vi "Verify Password.vi"(8 "error in (no error)":errorcluster) -> (0 "error out":errorcluster, 3 "Verified?":bool)   [LabVIEW 2017]
uses:
  <vilib>/Utility/sysdir.llb/System Directory Type.ctl
  <vilib>/Utility/config.llb/Write Key (String).vi
  <vilib>/Utility/config.llb/NI_LVConfig.lvlib
panel:
  in  "Verify":string
  in  "Cancel":bool
  in  "Change PWD":bool
  in  "Continue":bool
  in  "Password":string
  # "Administrative Password Management"
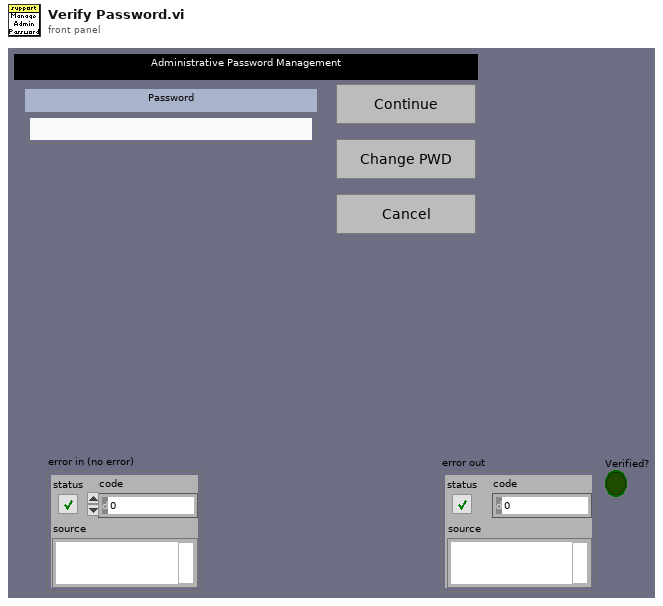
[diagram p1: front panel]
types:
  T1 = typedef "System Directory Type.ctl" = i32
  T2 = typedef "NI_LVConfig.lvlib/Config Data RefNum.ctl" = refnum<k1>
  T3 = enum8{"Enabled", "Disabled", "Disabled and Grayed Out"}
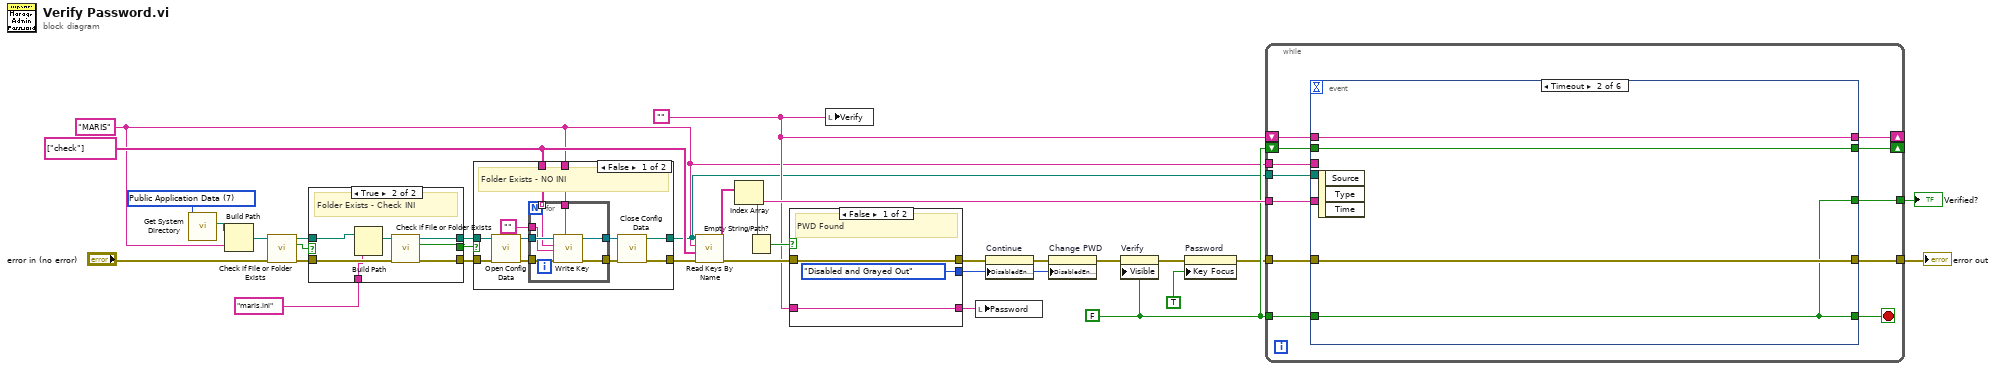
[diagram p0: block diagram]
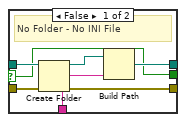
[diagram p3: hidden frame]
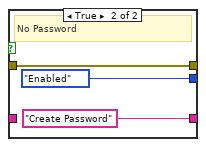
[diagram p4: hidden frame]
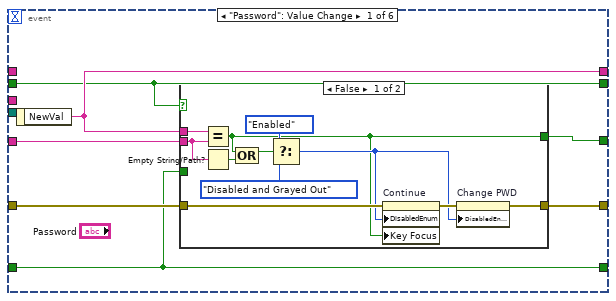
[diagram p5: hidden frame]
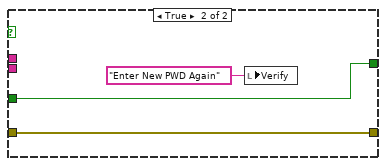
[diagram p6: hidden frame]
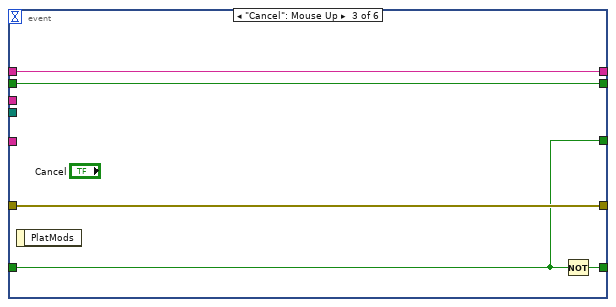
[diagram p7: hidden frame]
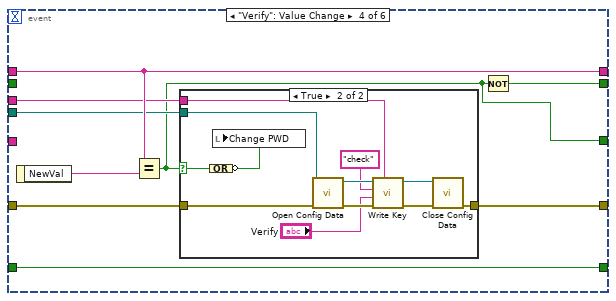
[diagram p8: hidden frame]
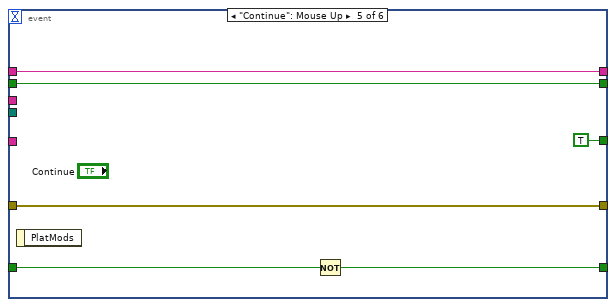
[diagram p10: hidden frame]
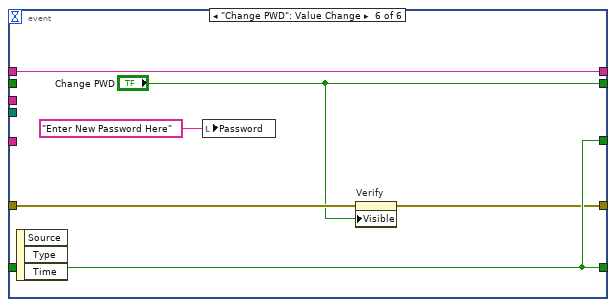
[diagram p11: hidden frame]
diagram:
  w4 = "MARIS" ("name or relative path")
  w18 = T1 7 items=["User Home"=0, "User Desktop"=1, "User Documents"=2, "User Application Data"=3, "User Preferences"=4, "User Temporary"=5, "Public Documents"=6, "Public Application Data"=7, "Public Preferences"=8, "Public Cache"=13, "System Core Libraries"=9, "System Installed Libraries"=10, "Application Files"=11, "Boot Volume Root"=12] ("system directory type")
  w21 = ""
  w7 = string[] ["check"] ("Search Keys")
  w19 = FALSE
  n1 = call <vilib>:"Get System Directory.vi"("system directory type"=w18) -> ("system directory"=w17:path)  [unwired: 10 in]
  n2 = Build Path(base path=w17, name or relative path=w4) -> (appended path=w16:path)
  n3 = call <vilib>:"Check if File or Folder Exists.vi"("error in (no error)"="error in (no error)", "path"=w16) -> ("error out"=w15:errorcluster, "file or folder exists?"=w13:bool, "dup path"=w14:path)  [unwired: 7 in]
  n4 = case shown="True" w13 {
    selector: w13 -> [w32 _]
    tunnel: w15 -> [w38 w45]
    tunnel: w14 -> [w37 w43]
    tunnel: [w34 w44] -> w10
    tunnel: [w33 w39] -> w8
    tunnel: "maris.ini" -> [w35 w42]
    tunnel: [w32 w40] -> w9
    frame False {
      # "No Folder - No INI File"
      n5 = Create Folder(path (use dialog)=w37, error in=w38) -> (created path=w36:path, error out=w34:errorcluster)  [unwired: 1 in, 1 out]
      n6 = Build Path(base path=w36, name or relative path=w35) -> (appended path=w33:path)
    }
    frame True {
      # "Folder Exists - Check INI"
      n7 = Build Path(base path=w43, name or relative path=w42) -> (appended path=w41:path)
      n8 = call <vilib>:"Check if File or Folder Exists.vi"("error in (no error)"=w45, "path"=w41) -> ("error out"=w44:errorcluster, "file or folder exists?"=w40:bool, "dup path"=w39:path)  [unwired: 7 in]
    }
  }
  n9 = case shown="False" w9 {
    tunnel: w10 -> [w52 w64]
    tunnel: w8 -> [w51 w65]
    tunnel: w4 -> [w50 _]
    tunnel: w7 -> [w49 _]
    tunnel: [w47 w64] -> w6
    tunnel: [w46 w65] -> w5
    frame False {
      # "Folder Exists - NO INI"
      n10 = call <vilib>:"Open Config Data.vi"("error in (no error)"=w52, "configuration file path"=w51) -> ("error out"=w53:errorcluster, "refnum"=w54:T2)  [unwired: 7 in, 1 out]
      n11 = for {
        tunnel: [w63] -> w56
        tunnel: [w62] -> w55
        tunnel: w54 -> [w61]
        tunnel: w53 -> [w60]
        tunnel: w50 -> [w59]
        tunnel: w49 -> [w58] mode=indexing
        tunnel: "" -> [w57]
        n12 = call-poly <vilib>:"Write Key.vi"("section"=w59, "error in (no error)"=w60, "value"=w57, "key"=w58, "refnum"=w61) -> ("error out"=w62:errorcluster, "refnum out"=w63:T2)  [unwired: 4 in, 1 out]
      }
      n13 = call <vilib>:"Close Config Data.vi"("error in (no error)"=w55, "refnum"=w56) -> ("error out"=w47:errorcluster, "file path"=w46:path)  [unwired: 8 in]
    }
    frame True {
      # "Folder and INI Exist"
    }
  }
  n14 = call "Read Keys By Name.vi"("error in (no error)"=w6, "Search Keys"=w7, "section"=w4, "Hardware INI Path"=w5) -> ("error out"=w28:errorcluster, "Key Data"=w31:string[])  [unwired: 6 in]
  n15 = Index Array(array=w31) -> (element=w29:string)  [unwired: 1 in]
  n16 = Empty String/Path?(string/path=w29) -> (empty?=w27:bool)
  n17 = case shown="False" w27 {
    tunnel: w28 -> [w68 w71]
    tunnel: [w68 w71] -> w23
    tunnel: [T3."Disabled and Grayed Out" ("Disabled") T3."Enabled" ("Disabled")] -> w22
    tunnel: [w66 "Create Password" ("Password")] -> w25
    tunnel: w21 -> [w66 _]
    frame False {
      # "PWD Found"
    }
    frame True {
      # "No Password"
    }
  }
  n18 = local write "Verify"(w21) -> ()
  n19 = local write "Password"(w25) -> ()
  n20 = property on="Continue" class="Bool"(error in=w23, "DisabledEnum"=w22) -> (error out=w24:errorcluster)  [unwired: 1 in, 1 out]
  n21 = property on="Change PWD" class="Bool (strict)"(error in=w24, "DisabledEnum"=w22) -> (error out=w20:errorcluster)  [unwired: 1 in, 1 out]
  n22 = property on="Verify" class="Str"(error in=w20, "Visible"=w19) -> (error out=w2:errorcluster)  [unwired: 1 in, 1 out]
  n23 = property on="Password" class="Str"(error in=w2, "Key Focus"=TRUE) -> (error out=w3:errorcluster)  [unwired: 1 in, 1 out]
  n24 = while {
    tunnel: w19 -> [w83]
    tunnel: w3 -> [w81]
    tunnel: w29 -> [w80]
    tunnel: [w79] -> w30
    tunnel: [w78] -> w26
    shift-right: [w77] -> _
    shift-left: w21 -> [w76]
    tunnel: w5 -> [w75]
    tunnel: w4 -> [w74]
    shift-right: [w73] -> _
    shift-left: w19 -> [w72]
    stop <- w82 stop-if-true
    n25 = event shown="[1] Timeout" {
      selector: _ -> [_ _ _ _ _ _]
      dyn-events: _ -> [_ _ _ _ _ _]
      timeout: _ -> [_ _ _ _ _ _]
      tunnel: w83 -> [w84 w105 w111 w115 w140 w147]
      tunnel: [w84 w105 w113 w115 w138 w147] -> w82
      tunnel: w81 -> [w90 w106 w112 w120 w141 w145]
      tunnel: w80 -> [w88 _ _ _ _ _]
      tunnel: [w89 w106 w112 w119 w141 w144] -> w79
      tunnel: [w85 w105 w111 w114 TRUE w147] -> w78
      tunnel: [w87 w108 w110 w122 w139 w146] -> w77
      tunnel: w76 -> [_ w108 w110 w122 w139 w146]
      tunnel: w75 -> [_ _ _ w117 _ _]
      tunnel: w74 -> [_ _ _ w116 _ _]
      tunnel: [w86 w107 w109 w118 w137 "Change PWD"] -> w73
      tunnel: w72 -> [w86 w107 w109 _ w137 _]
      event "Password": Value Change {
        n26 = event-data() -> ("NewVal"=w87:string)  [unwired: 1 in]
        n27 = case shown="False" w86 {
          tunnel: w90 -> [w101 w104]
          tunnel: [w96 w104] -> w89
          tunnel: w88 -> [w95 _]
          tunnel: w87 -> [w92 _]
          tunnel: [w91 w103] -> w85
          tunnel: w84 -> [_ w103]
          frame False {
            n28 = Equal?(x=w92, y=w95) -> (x = y?=w91:bool)
            n29 = Empty String/Path?(string/path=w95) -> (empty?=w93:bool)
            n30 = Compound Arithmetic op=OR(w91, w93) -> (w94:bool)
            n31 = Select(t=T3."Enabled" ("Disabled"), s=w94, f=T3."Disabled and Grayed Out") -> (s? t:f=w98:T3)
            n32 = property on="Continue" class="Bool"(error in=w101, "DisabledEnum"=w98, "Key Focus"=w91) -> (error out=w100:errorcluster)  [unwired: 1 in, 1 out]
            n33 = property on="Change PWD" class="Bool (strict)"(error in=w100, "DisabledEnum"=w98) -> (error out=w96:errorcluster)  [unwired: 1 in, 1 out]
          }
          frame True {
            n34 = local write "Verify"("Enter New PWD Again" ("Verify")) -> ()
          }
        }
      }
      event Timeout {
        n35 = event-data() -> ()  [unwired: 1 in, 3 out]
      }
      event "Cancel": Mouse Up {
        n36 = event-data() -> ()  [unwired: 1 in, 1 out]
        n37 = Not(x=w111) -> (.not. x?=w113:bool)
      }
      event "Verify": Value Change {
        n38 = event-data() -> ("NewVal"=w121:string)  [unwired: 1 in]
        n39 = Equal?(x=w122, y=w121) -> (x = y?=w114:bool)
        n40 = case shown="True" w114 {
          selector: w114 -> [_ w125]
          tunnel: w120 -> [w123 w129]
          tunnel: [w123 w128] -> w119
          tunnel: w117 -> [_ w127]
          tunnel: w116 -> [_ w126]
          frame False {
          }
          frame True {
            n41 = Compound Arithmetic op=OR(w125) -> (invert w124:bool)
            n42 = local write "Change PWD"(w124) -> ()
            n43 = call <vilib>:"Open Config Data.vi"("error in (no error)"=w129, "configuration file path"=w127) -> ("error out"=w132:errorcluster, "refnum"=w133:T2)  [unwired: 7 in, 1 out]
            n44 = call-poly <vilib>:"Write Key.vi"("section"=w126, "error in (no error)"=w132, "value"="Verify", "key"="check", "refnum"=w133) -> ("error out"=w134:errorcluster, "refnum out"=w135:T2)  [unwired: 4 in, 1 out]
            n45 = call <vilib>:"Close Config Data.vi"("error in (no error)"=w134, "refnum"=w135) -> ("error out"=w128:errorcluster)  [unwired: 8 in, 1 out]
          }
        }
        n46 = Not(x=w114) -> (.not. x?=w118:bool)
      }
      event "Continue": Mouse Up {
        n47 = event-data() -> ()  [unwired: 1 in, 1 out]
        n48 = Not(x=w140) -> (.not. x?=w138:bool)
      }
      event "Change PWD": Value Change {
        n49 = event-data() -> ()  [unwired: 1 in, 3 out]
        n50 = local write "Password"("Enter New Password Here" ("Password")) -> ()
        n51 = property on="Verify" class="Str"(error in=w145, "Visible"="Change PWD") -> (error out=w144:errorcluster)  [unwired: 1 in, 1 out]
      }
    }
  }
  "error out" <- w30
  "Verified?" <- w26
